vi "Gaussian Window.vi"   [LabVIEW 2010, in "NI_AALPro.lvlib"]
doc: "Applies an asymmetrical Gaussian window to the input sequence <B>X</B>. Wire data to the <B>X</B> input to determine the polymorphic instance to use or manually select the instance."
uses:
  NI_AALPro.lvlib
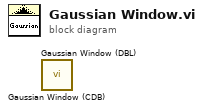
[diagram p0: block diagram]
diagram:
  n1 = call "Gaussian Window (CDB).vi"() -> ()  [unwired: 10 in, 2 out]
  n2 = call "Gaussian Window (DBL).vi"() -> ()  [unwired: 10 in, 2 out]
